vi "AskBandName.vi"(7 "Filters":string, 8 "error in (no error)":errorcluster, 10 "Default name":string) -> (0 "error out":errorcluster, 1 "List":string, 2 "OK":bool)   [LabVIEW 2022 SP3]
uses:
  <vilib>/Utility/miscctls.llb/LVSelectionTypeDef.ctl
panel:
  out "String":string="Enter the name of the new list."
  in  "Cancel":bool
  in  "OK2":bool
  in  "Band File":string caption="List"
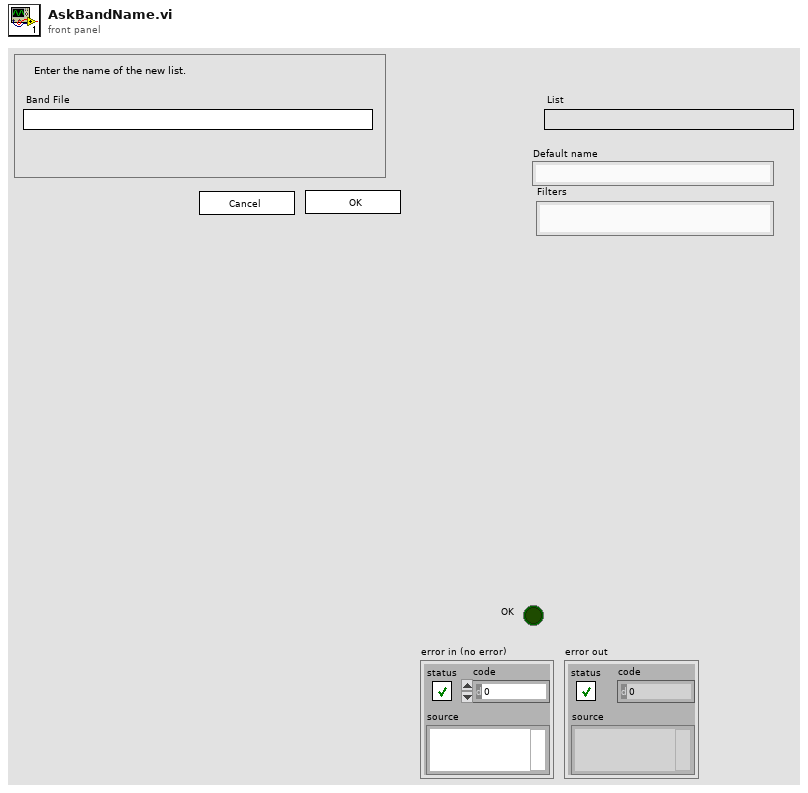
[diagram p1: front panel]
types:
  T1 = typedef "LVSelectionTypeDef.ctl" = cluster{"Selection Start":u32, "Selection End":u32}
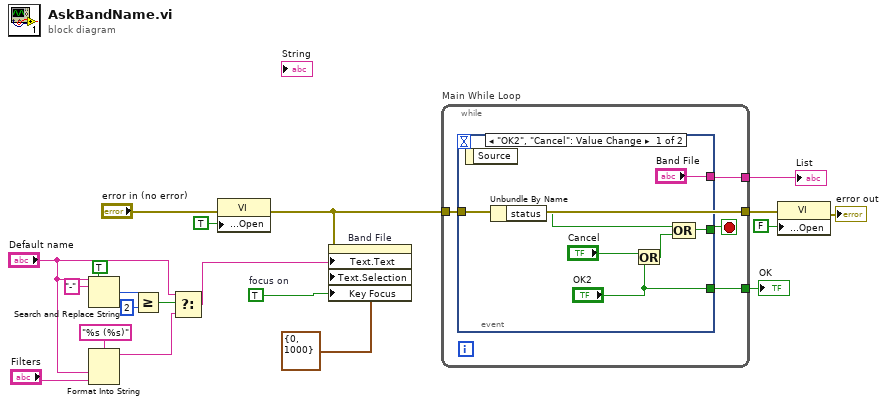
[diagram p0: block diagram]
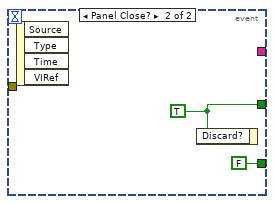
[diagram p2: hidden frame]
diagram:
  w14 = TRUE  # focus on
  n1 = Search and Replace String(replace all?=TRUE ("replace all? (F)"), input string="Default name", search string="-") -> (number of replacements=w9:i32)  [unwired: 5 in, 3 out]
  n2 = Format Into String(format string="%s (%s)", "Default name", "Filters") -> (resulting string=w1:string)  [unwired: 2 in, 1 out]
  n3 = Greater Or Equal?(x=w9, y=2) -> (x >= y?=w7:bool)
  n4 = Select(t="Default name", s=w7, f=w1) -> (s? t:f=w6:string)
  n5 = property class="VI"(error in="error in (no error)", "Front Panel Window:Open"=TRUE) -> (error out=w19:errorcluster)  [unwired: 1 in, 1 out]
  n6 = property on="Band File" class="Str"(error in=w19, "Text.Text"=w6, "Text.Selection"=T1 {"Selection Start"=0, "Selection End"=1000}, "Key Focus"=w14) -> ()  [unwired: 1 in, 2 out]
  n7 = while "Main While Loop" {
    tunnel: [w24] -> w20
    tunnel: w19 -> [w23]
    tunnel: [w23] -> w18
    tunnel: [w21] -> w15
    stop <- w22 stop-if-true
    n8 = event shown="[0] \"OK2\", \"Cancel\": Value Change" {
      selector: _ -> [_ _]
      dyn-events: _ -> [_ _]
      timeout: _ -> [_ _]
      tunnel: ["OK2" FALSE ("OK2")] -> w24
      tunnel: [w30 w33] -> w22
      tunnel: w23 -> [w29 _]
      tunnel: ["Band File" _] -> w21
      event "OK2", "Cancel": Value Change {
        n9 = event-data() -> ()  [unwired: 1 in, 1 out]
        n10 = Unbundle By Name(w29) -> ("status"=w27:bool)
        n11 = Or(x="Cancel", y="OK2") -> (x .or. y?=w28:bool)
        n12 = Compound Arithmetic op=OR(w27, w28) -> (w30:bool)
      }
      event Panel Close? {
        w33 = TRUE ("Discard?")
        n13 = event-data() -> ()  [unwired: 1 in, 4 out]
        n14 = event-data("Discard?"=w33) -> ()  [unwired: 1 in, 1 out]
      }
    }
  }
  "OK" <- w20
  "List" <- w15
  n15 = property class="VI"(error in=w18, "Front Panel Window:Open"=FALSE) -> (error out=→"error out":errorcluster)  [unwired: 1 in, 1 out]
